vi "initialize HW.vi"(8 "error in":errorcluster, 11 "DAQ Config":T1) -> (0 "error out":errorcluster, 3 "DAQ Config out":T1)   [LabVIEW 2017]
uses:
  Control/Config chanel.ctl
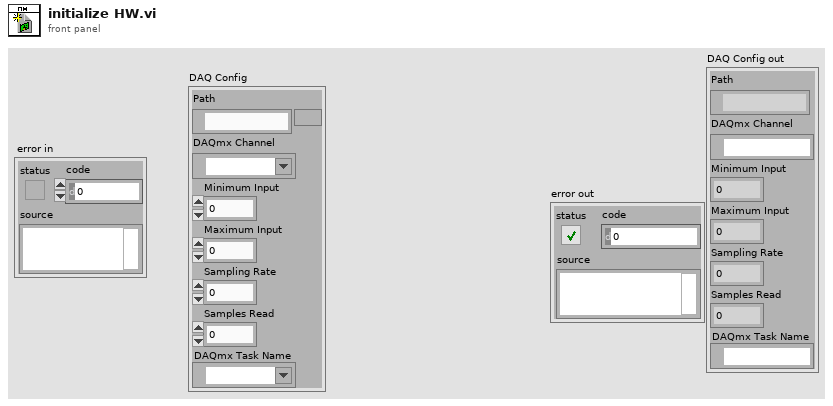
[diagram p1: front panel]
types:
  T1 = typedef "Config chanel.ctl" = cluster{"Path":path, "DAQmx Channel":tag, "Minimum Input":dbl, "Maximum Input":dbl, "Sampling Rate":dbl, "Samples Read":dbl, "DAQmx Task Name":refnum<k21>}
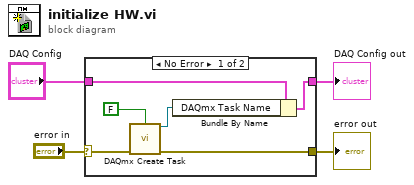
[diagram p0: block diagram]
diagram:
  n1 = case shown="No Error" "error in" {
    selector: "error in" -> [w7 w12]
    tunnel: [w6 w12] -> w3
    tunnel: "DAQ Config" -> [w9 w11]
    tunnel: [w5 w11] -> w1
    frame No Error {
      n2 = call <vilib>:"DAQmx Create Task.vi"("auto cleanup"=FALSE, "error in"=w7) -> ("task out"=w8:refnum<k21>, "error out"=w6:errorcluster)  [unwired: 12 in]
      n3 = Bundle By Name(cluster=w9, "DAQmx Task Name"=w8) -> (w5:T1)
    }
    frame Error {
    }
  }
  "error out" <- w3
  "DAQ Config out" <- w1
